vi "Write State.vi"(8 "error in (no error)":errorcluster, 10 "State":refnum<class "State Pattern.lvclass">, 11 "B Context State in":refnum<class "B Context State.lvclass">) -> (0 "error out":errorcluster, 3 "B Context State out":refnum<class "B Context State.lvclass">)   [LabVIEW 2021, in "B Context State.lvclass"]
uses:
  B Context State.lvclass
  State Pattern/State Pattern.lvclass
  B Context State.lvclass/B Context State.ctl
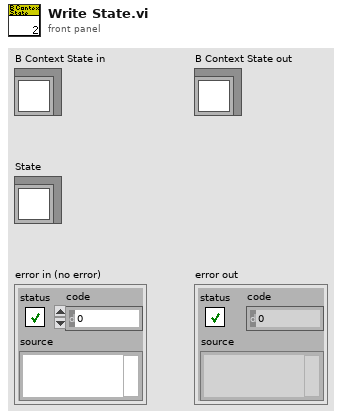
[diagram p1: front panel]
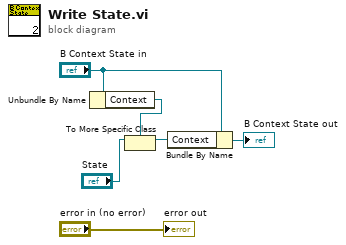
[diagram p0: block diagram]
diagram:
  n1 = Unbundle By Name("B Context State in") -> ("Context"=w1:refnum<class "Context.lvclass">)
  n2 = To More Specific Class(target class=w1, reference="State") -> (specific class reference=w4:refnum<class "Context.lvclass">)  [unwired: 1 in, 1 out]
  n3 = Bundle By Name(cluster="B Context State in", "Context"=w4) -> (→"B Context State out":refnum<class "B Context State.lvclass">)
  "error out" <- "error in (no error)"
